vi "PH_TKTDS-30xx.Configure Hardware.vi"(0 "i ref in":refnum<vi>, 2 "Channels Sets":T3(array[cluster]) {"Chan Settings"."Vertical Offset" format="%#_6p"; "Chan Settings"."Vertical Range" items=["1mV"=0.001, "2mV"=0.002, "5mV"=0.005, "10mV"=0.01, "20mV"=0.02, "50mV"=0.05, "100mV"=0.1, "200mV"=0.2, "500mV"=0.5, "1V"=1.0]; "Chan Settings"."Probe Attenuation" format="%#.2f"}, 3 "Trigger Settings":T5={"Source"="CH1", "Slope"=0, "Level [V]"=0.0} {"Level [V]" format="%#_6p"}, 4 "Acqu Settings":T4={"Time base"=2e-07, "Record Length"=10000, "Start Time"=0.0, "Type"=0, "Continuous"=FALSE} {"Start Time" format="%#_12p"; "Record Length" items=["500"=500, "10000"=10000]; "Time base" items=["2ns"=2e-09, "4ns"=4e-09, "10ns"=1e-08, "20ns"=2e-08, "40ns"=4e-08, "100ns"=1e-07, "200ns"=2e-07, "400ns"=4e-07, "1µs"=1e-06, "2µs"=2e-06, "4µs"=4e-06, "10µs"=1e-05, "20µs"=2e-05, "40µs"=4e-05, "100µs"=0.0001, "200µs"=0.0002, "400µs"=0.0004, "1ms"=0.001, "2ms"=0.002, "10ms"=0.01, "20ms"=0.02, "40ms"=0.04, "100ms"=0.1, "200ms"=0.2, "400ms"=0.4, "1s"=1.0, "2s"=2.0, "4s"=4.0, "10s"=10.0]}, 5 "error in":errorcluster) -> (14 "i ref out":refnum<vi>, 19 "error out":errorcluster)   [LabVIEW 2014, in "PH_TKTDS-30xx.lvlib"]
doc: "This VI sets the hardware."
uses:
  PH_TKTDS-30xx.lvlib
  PH_TKTDS-30xx.Trigger Config.ctl
  PH_TKTDS-30xx.Acquisition Config.ctl
  PH_TKTDS-30xx.Channel Config.ctl
  PH_TKTDS-30xx.Waveform Limits.ctl
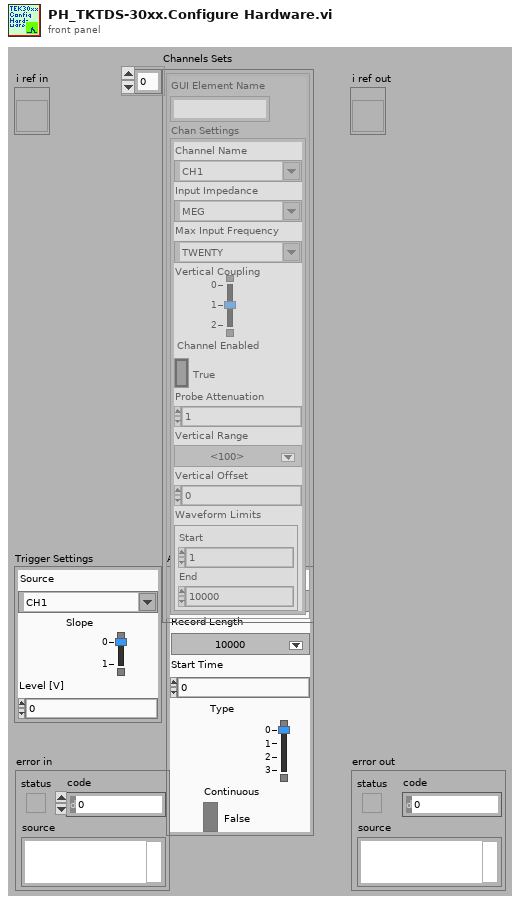
[diagram p1: front panel]
types:
  T1 = typedef "PH_TKTDS-30xx.lvlib/PH_TKTDS-30xx.Channel Config.ctl" = cluster{"Channel Name":string, "Input Impedance":string, "Max Input Frequency":string, "Vertical Coupling":i32, "Channel Enabled":bool, "Probe Attenuation":dbl, "Vertical Range":dbl, "Vertical Offset":dbl, "Waveform Limits":T2}
  T2 = typedef "PH_TKTDS-30xx.lvlib/PH_TKTDS-30xx.Waveform Limits.ctl" = cluster{"Start":i32, "End":i32}
  T3 = cluster{"GUI Element Name":string, "Chan Settings":T1}[]
  T4 = typedef "PH_TKTDS-30xx.lvlib/PH_TKTDS-30xx.Acquisition Config.ctl" = cluster{"Time base":dbl, "Record Length":u16, "Start Time":dbl, "Type":i32, "Continuous":bool}
  T5 = typedef "PH_TKTDS-30xx.lvlib/PH_TKTDS-30xx.Trigger Config.ctl" = cluster{"Source":string, "Slope":i32, "Level [V]":dbl}
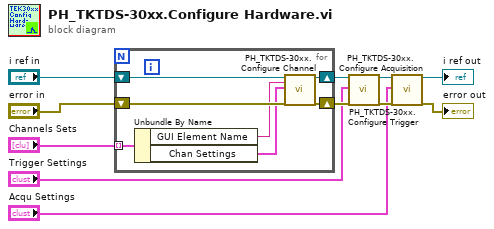
[diagram p0: block diagram]
diagram:
  n1 = for {
    shift-right: [w15] -> w8
    shift-left: "error in" -> [w18]
    shift-right: [w17] -> w9
    shift-left: "i ref in" -> [w16]
    tunnel: "Channels Sets" -> [w14] mode=indexing
    n2 = Unbundle By Name(w14) -> ("GUI Element Name"=w13:string, "Chan Settings"=w12:T1)
    n3 = call "PH_TKTDS-30xx.Configure Channel.vi"("i ref in"=w16, "GUI Element Name"=w13, "Channel Configuration"=w12, "error IO"=w18) -> ("i ref out"=w17:refnum<vi>, "error out"=w15:errorcluster)  [unwired: 14 in]
  }
  n4 = call "PH_TKTDS-30xx.Configure Trigger.vi"("i ref in"=w9, "Trigger Configuration"="Trigger Settings", "error IO"=w8) -> ("i ref out"=w11:refnum<vi>, "error out"=w10:errorcluster)  [unwired: 15 in]
  n5 = call "PH_TKTDS-30xx.Configure Acquisition.vi"("i ref in"=w11, "Acquisition Configuration"="Acqu Settings", "error IO"=w10) -> ("i ref out"=→"i ref out":refnum<vi>, "error out"=→"error out":errorcluster)  [unwired: 15 in]
